vi "capsule detect.vi"() -> ()   [LabVIEW 2021]
uses:
  <vilib>/vision/NI_Vision_Development_Module.lvlib
panel:
  out "Image":T1(plugin-control)
  in  "等待时间（毫秒）":u32=1000
  out "pass?":bool
  in  "stop":bool
  in  "Search Strategy":u32(ring)=1 items=["Conservative", "Balance", "Aggressive", "Very Aggressive"]
  in  "Color Sensitivity":u32(ring)=1 items=["Low Sensitivity", "Medium Sensitivity", "High Sensitivity"]
  out "Matches":i32
  out "status":T2(ring)
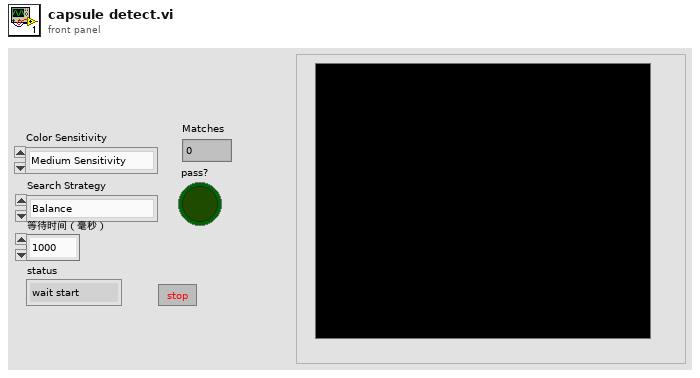
[diagram p1: front panel]
types:
  T1 = typedef "IMAQ Image.ctl" = refnum<image>
  T2 = enum16{"wait start", "learn", "setup match", "match", "exit"}
  T3 = typedef "Image Type" = u32
  T4 = cluster{"Position":cluster{"x":sgl, "y":sgl}, "Angle":sgl, "Scale":sgl, "Score":sgl, "Bounding Box":cluster{"x":sgl, "y":sgl}[]}[]
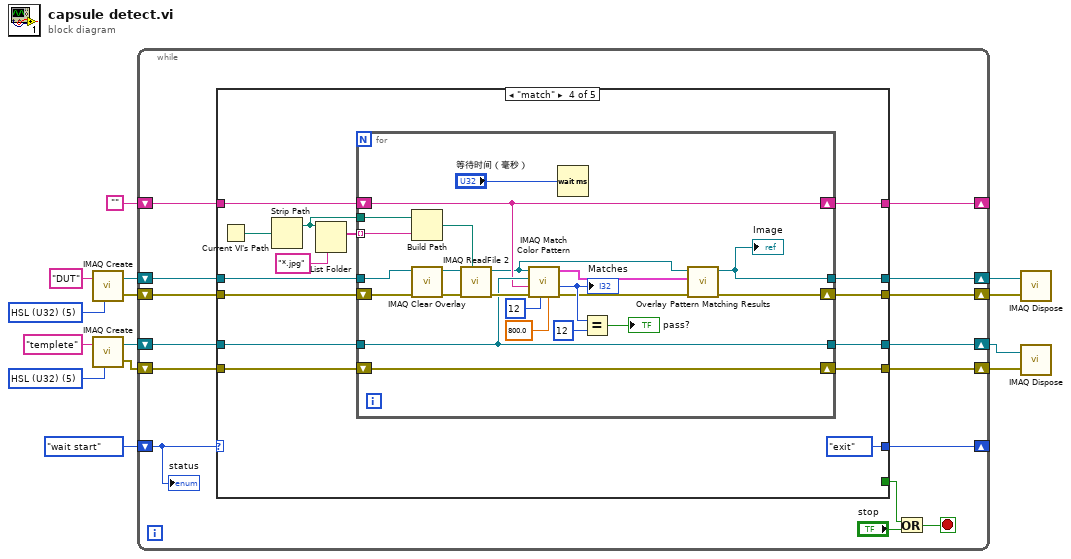
[diagram p0: block diagram]
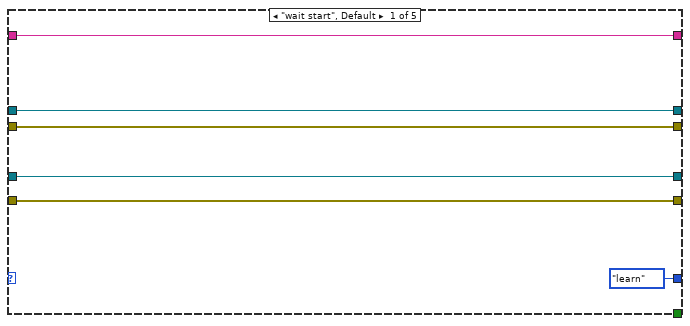
[diagram p2: hidden frame]
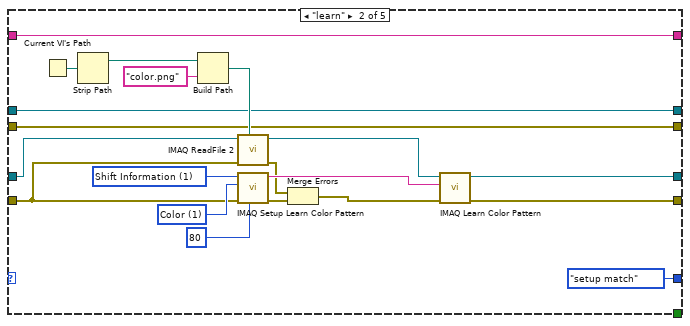
[diagram p3: hidden frame]
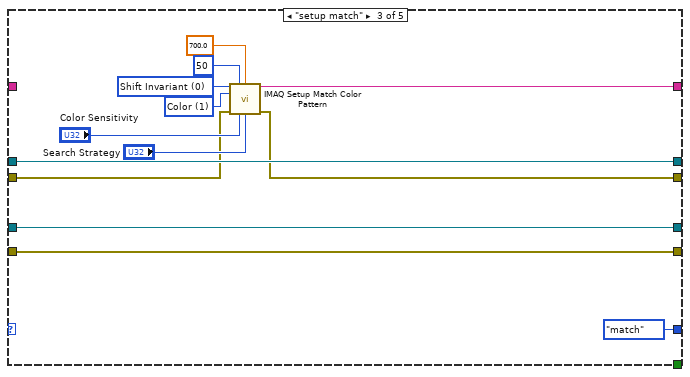
[diagram p4: hidden frame]
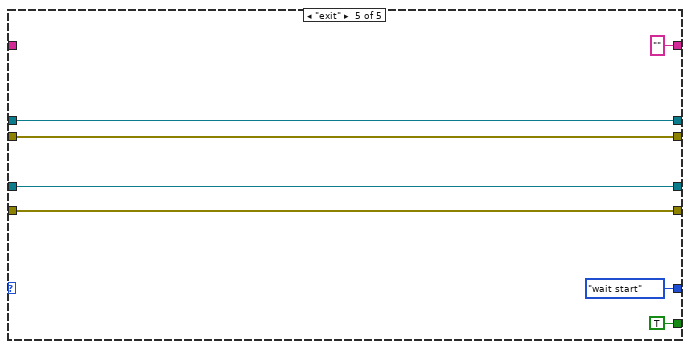
[diagram p5: hidden frame]
diagram:
  w9 = T3 5 items=["Grayscale (U8)", "Grayscale (I16)", "Grayscale (SGL)", "Complex (CSG)", "RGB (U32)", "HSL (U32)", "RGB (U64)", "Grayscale (U16)"] ("Image Type")
  w14 = T3 5 items=["Grayscale (U8)", "Grayscale (I16)", "Grayscale (SGL)", "Complex (CSG)", "RGB (U32)", "HSL (U32)", "RGB (U64)", "Grayscale (U16)"] ("Image Type")
  n1 = call "IMAQ Create"("Image Name"="DUT", "Image Type"=w9) -> ("New Image"=w8:T1, "error out"=w7:errorcluster)  [unwired: 3 in]
  n2 = call "IMAQ Create"("Image Name"="templete", "Image Type"=w14) -> ("New Image"=w12:T1, "error out"=w11:errorcluster)  [unwired: 3 in]
  n3 = while {
    shift-right: [w28] -> w4
    shift-left: w11 -> [w29]
    shift-right: [w27] -> w3
    shift-left: w12 -> [w26]
    shift-right: [w25] -> _
    shift-left: "" -> [w24]
    shift-right: [w20] -> w5
    shift-left: w8 -> [w23]
    shift-right: [w21] -> w6
    shift-left: w7 -> [w22]
    shift-right: [w18] -> _
    shift-left: T2."wait start" ("status") -> [w19]
    stop <- w15 stop-if-true
    n4 = case shown="\"match\"" w19 {
      tunnel: w29 -> [w31 w40 w67 w76 w108]
      tunnel: [w31 w47 w67 w75 w108] -> w28
      tunnel: [w32 w46 w68 w74 w109] -> w27
      tunnel: w26 -> [w32 w45 w68 w77 w109]
      tunnel: [w35 w43 w60 w72 "" ("Match Color Pattern Setup Data")] -> w25
      tunnel: w24 -> [w35 w43 _ w78 _]
      tunnel: w23 -> [w34 w41 w59 w80 w110]
      tunnel: w22 -> [w33 w42 w57 w79 w111]
      tunnel: [w33 w42 w56 w73 w111] -> w21
      tunnel: [w34 w41 w59 w70 w110] -> w20
      tunnel: [_ _ _ _ TRUE] -> w16
      tunnel: [T2."learn" ("status") T2."setup match" ("status") T2."match" ("status") T2."exit" ("status") T2."wait start" ("status")] -> w18
      frame "wait start", Default {
      }
      frame "learn" {
        w54 = u32 1 items=["Color and Shape", "Color", "Shape "] ("Feature Mode")
        w55 = u32 1 items=["All", "Shift Information", "Rotation Information"] ("Learn Mode")
        n5 = Current VI's Path() -> (path=w52:path)
        n6 = Strip Path(path=w52) -> (stripped path=w51:path)  [unwired: 1 out]
        n7 = Build Path(base path=w51, name or relative path="color.png") -> (appended path=w44:path)
        n8 = call "IMAQ ReadFile 2"("File Path"=w44, "error in (no error)"=w40, "Image"=w45) -> ("error out"=w36:errorcluster, "Image Out"=w49:T1)  [unwired: 4 in, 3 out]
        n9 = call "IMAQ Setup Learn Color Pattern"("Saturation Threshold"=80, "error in (no error)"=w40, "Feature Mode"=w54, "Learn Mode"=w55) -> ("error out"=w38:errorcluster, "Learn Color Pattern Setup Data"=w48:string)  [unwired: 6 in]
        n10 = Merge Errors(w36, w38) -> (w37:errorcluster)
        n11 = call "IMAQ Learn Color Pattern"("error in (no error)"=w37, "Learn Color Pattern Setup Data"=w48, "Image"=w49) -> ("error out"=w47:errorcluster, "Template Image Out"=w46:T1)  [unwired: 7 in]
      }
      frame "setup match" {
        w63 = u32 1 items=["Color and Shape", "Color", "Shape"] ("Match Feature Mode")
        w66 = u32 0 items=["Shift Invariant", "Rotation Invariant"] ("Match Mode")
        n12 = call "IMAQ Setup Match Color Pattern"("Match Mode"=w66, "Minimum Contrast"=50, "Color Score Weight"=sgl 700.0, "Match Feature Mode"=w63, "error in (no error)"=w57, "Color Sensitivity"="Color Sensitivity", "Search Strategy"="Search Strategy") -> ("Match Color Pattern Setup Data"=w60:string, "error out"=w56:errorcluster)  [unwired: 7 in]
      }
      frame "match" {
        n13 = Current VI's Path() -> (path=w81:path)
        n14 = Strip Path(path=w81) -> (stripped path=w69:path)  [unwired: 1 out]
        n15 = List Folder(path=w69, pattern="*.jpg" ("类型")) -> (filenames=w82:string[])  [unwired: 2 in, 3 out]
        n16 = for {
          tunnel: w82 -> [w104] mode=indexing
          tunnel: w69 -> [w105]
          tunnel: w80 -> [w86]
          tunnel: w77 -> [w97]
          shift-right: [w101] -> w75
          shift-left: w76 -> [w101]
          shift-right: [w91] -> w73
          shift-left: w79 -> [w88]
          tunnel: [w97] -> w74
          shift-right: [w96] -> w72
          shift-left: w78 -> [w96]
          tunnel: [w84] -> w70
          n17 = Build Path(base path=w105, name or relative path=w104) -> (appended path=w103:path)
          n18 = call "IMAQ Clear Overlay"("error in (no error)"=w88, "Image"=w86) -> ("error out"=w87:errorcluster, "Image Out"=w85:T1)  [unwired: 8 in]
          n19 = call "IMAQ ReadFile 2"("File Path"=w103, "error in (no error)"=w87, "Image"=w85) -> ("error out"=w102:errorcluster, "Image Out"=w89:T1)  [unwired: 4 in, 3 out]
          n20 = call "IMAQ Match Color Pattern"("Minimum Match Score"=sgl 800.0, "Number of Matches Requested"=12, "error in (no error)"=w102, "Match Color Pattern Setup Data"=w96, "Template Image"=w97, "Image"=w89) -> ("error out"=w92:errorcluster, "Number of Matches"=w95:i32, "Matches"=w90:T4)  [unwired: 3 in]
          "Matches" <- w95
          n21 = Wait (ms)(milliseconds to wait="等待时间（毫秒）") -> ()  [unwired: 1 out]
          n22 = Equal?(x=w95, y=12) -> (x = y?=→"pass?":bool)
          n23 = call "Overlay Pattern Matching Results.vi"("error in"=w92, "Matches"=w90, "Image"=w89) -> ("error out"=w91:errorcluster, "Image Out"=w84:T1)  [unwired: 7 in]
          "Image" <- w84
        }
      }
      frame "exit" {
      }
    }
    n24 = Or(x=w16, y="stop") -> (x .or. y?=w15:bool)
    "status" <- w19
  }
  n25 = call "IMAQ Dispose"("Image"=w5, "error in (no error)"=w6) -> ()  [unwired: 4 in, 1 out]
  n26 = call "IMAQ Dispose"("Image"=w3, "error in (no error)"=w4) -> ()  [unwired: 4 in, 1 out]
